vi "Print Options Read 2.vi"(4 "error in (no error)":errorcluster, 6 "Container State":T2, 7 "Display State In":T1) -> (0 "error out":errorcluster, 2 "Value":refnum<k24>, 3 "Display State Out":T1)   [LabVIEW 2020, in "WebView2 Control.xctl"]
uses:
  WebView2 Control.xctl
  <vilib>/_xctls/Container State.ctl
  State.ctl
  Webview2 Lib/WebView2 Control Object/WebView2 Control.lvclass
  C:/Users/Simon/Documents/GitHub/LV-WebView2/Source/Libs/Microsoft.Web.WebView2.Core.dll
  Libs/Microsoft.Web.WebView2.Core.dll
  Webview2 Lib/WebView2 Control Object/Read Print Options.vi
  <vilib>/_xctls/XControlSupport.lvlib
panel:
  # "Replace the Value Indicator below with an Indicator of desired type.\nDo not remove this Indicator or the others from the connector pane. \nDo not change the connector pane pattern.\nThe Value Indicator should always be the second terminal from top on the output side in the connector pane."
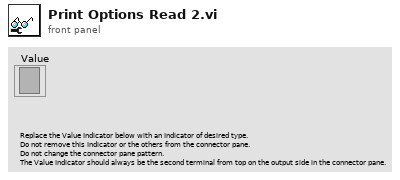
[diagram p1: front panel]
types:
  T1 = typedef "WebView2 Control.xctl/State.ctl" = cluster{"Control Object Ref":refnum<data-value>, "Used?":bool}
  T2 = typedef "XControlSupport.lvlib/Container State.ctl" = cluster{"Indicator?":bool, "Run Mode?":bool, " Refnum":refnum<vi>}
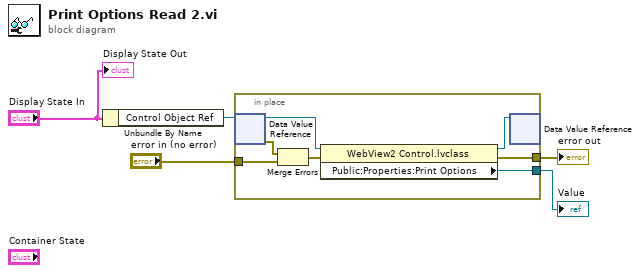
[diagram p0: block diagram]
diagram:
  n1 = Unbundle By Name("Display State In") -> ("Control Object Ref"=w5:refnum<data-value>)
  n2 = in-place {
    in-place-border: "error in (no error)" -> [w11]
    in-place-border: [w7] -> w2
    in-place-border: [w6] -> w1
    n3 = in-place-dvr #1(w5) -> (w10:refnum<class "WebView2 Control.lvclass">, w12:errorcluster)
    n4 = Merge Errors(w12, w11) -> (w9:errorcluster)
    n5 = property class="WebView2 Control.lvclass"(reference=w10, error in=w9) -> (reference out=w8:refnum<class "WebView2 Control.lvclass">, error out=w6:errorcluster, "Public:Properties:Print Options"=w7:refnum<k24>)
    n6 = in-place-dvr #1(w8) -> ()  [unwired: 2 out]
  }
  "error out" <- w1
  "Value" <- w2
  "Display State Out" <- "Display State In"
